vi "GetFilePaths.vi"(8 "error in (no error)":errorcluster, 11 "SaveForPrevious in":refnum<class "SaveForPrevious.lvclass">) -> (0 "error out":errorcluster, 1 "Destinations":path[](array[path]), 2 "Sources":path[](array[path]), 3 "SaveForPrevious out":refnum<class "SaveForPrevious.lvclass">)   [LabVIEW 2014, in "SaveForPrevious.lvclass"]
uses:
  SaveForPrevious.lvclass
  SaveForPrevious.lvclass/SaveForPrevious.ctl
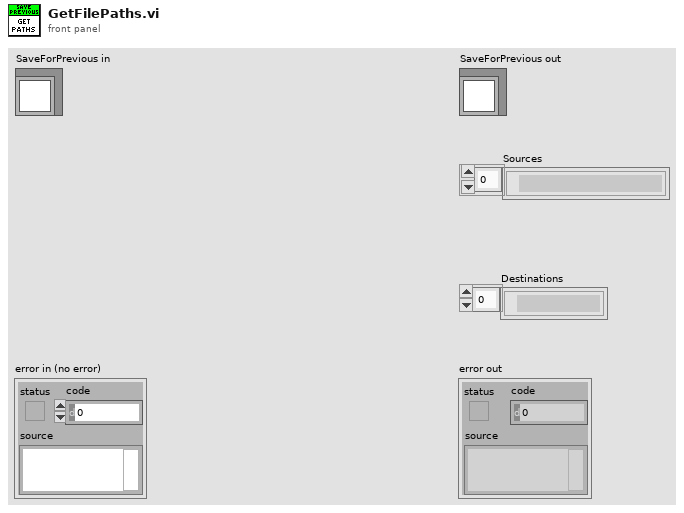
[diagram p1: front panel]
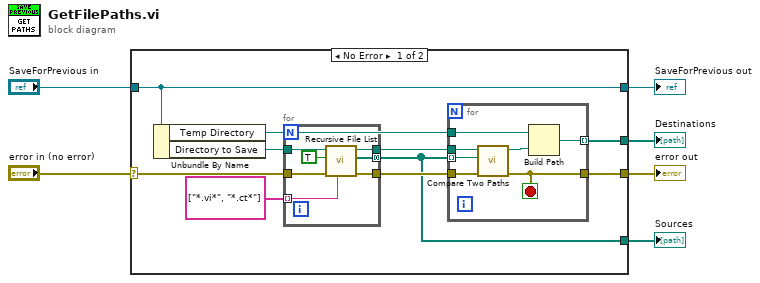
[diagram p0: block diagram]
diagram:
  n1 = case shown="No Error" "error in (no error)" {
    selector: "error in (no error)" -> [w14 w32]
    tunnel: [w12 w32] -> w5
    tunnel: [w8 w31] -> w3
    tunnel: "SaveForPrevious in" -> [w8 w31]
    tunnel: [w11 _] -> w2
    tunnel: [w10 _] -> w1
    frame No Error {
      n2 = Unbundle By Name(w8) -> ("Temp Directory"=w9:path, "Directory to Save"=w15:path)
      n3 = for {
        tunnel: [w18] -> w10 mode=concatenating
        tunnel: w15 -> [w21]
        tunnel: [w22] -> w16
        tunnel: w14 -> [w20]
        tunnel: [w19] -> w13
        tunnel: string[] ["*.vi*", "*.ct*"] -> [w17] mode=indexing
        n4 = call <vilib>:"Recursive File List.vi"("pattern"=w17, "error in (no error)"=w20, "Treat LLBs as Folders?"=TRUE, "Folder Path"=w21) -> ("error out"=w19:errorcluster, "All Files in Dir"=w18:path[], "dup Folder Path"=w22:path)  [unwired: 3 in, 2 out]
      }
      n5 = for {
        tunnel: w16 -> [w30]
        tunnel: w10 -> [w29] mode=indexing
        tunnel: w9 -> [w28]
        tunnel: [w26] -> w11 mode=indexing
        tunnel: w13 -> [w25]
        tunnel: [w24] -> w12
        stop <- w24 stop-if-true
        n6 = call <vilib>:"Compare Two Paths.vi"("error in (no error)"=w25, "Path 2"=w29, "Path 1"=w30) -> ("error out"=w24:errorcluster, "Relative Path from 1 to 2"=w27:path)  [unwired: 5 in, 2 out]
        n7 = Build Path(base path=w28, name or relative path=w27) -> (appended path=w26:path)
      }
    }
    frame Error {
    }
  }
  "error out" <- w5
  "SaveForPrevious out" <- w3
  "Destinations" <- w2
  "Sources" <- w1
